vi "Write Prev CCD Config.vi"(8 "error in (no error)":errorcluster, 10 "Prev CCD Config":T1={"PREAMP"=0, "READOUT_RATE"=0, "EM_GAIN"=2, "VERTICAL_SHIFT_SPEED"=0, "READ_MODE"=4, "FRAME_TRANSFER"=TRUE, "VERTICAL_CLOCK_VOLTAGE"=0, "ACQUISITION_MODE"=2, "AD_CHANNEL"=0, "EM_MODE"=0, "SHUTTER_TTL"=0, "SHUTTER_OPENING_TIME"=50, "SHUTTER_CLOSING_TIME"=50, "SHUTTER_MODE"=2, "TRIGGER_MODE"=0, "VBIN"=1, "INITIAL_LINE"=1, "INITIAL_COLUMN"=1, "FINAL_LINE"=1024, "FINAL_COLUMN"=1024, "HBIN"=1} {"TRIGGER_MODE" items=["Internal", "External", "N/A", "N/A_1", "N/A_2", "N/A_3", "External Start"]; "SHUTTER_MODE" items=["Auto", "Open", "Closed"]; "SHUTTER_TTL" items=["TTL Low", "TTL High"]; "EM_MODE" items=["Electron Multiplying", "Conventional"]; "ACQUISITION_MODE" items=["Single", "Accumulate", "Kinetic"]; "VERTICAL_CLOCK_VOLTAGE" items=["0", "+1", "+2", "+3", "+4"]; "READ_MODE" items=["Full Vertical Binning", "Multi-track", "Random-track", "Single-track", "Image"]; "VERTICAL_SHIFT_SPEED" items=["0.6", "1.13", "2.2", "4.33"]; "READOUT_RATE" items=["1 MHz", "0.1 MHz"]; "PREAMP" items=["Gain 1", "Gain 2"]}, 11 "Simulated_CCD_Camera in":refnum<class "Simulated Camera.lvclass">) -> (0 "error out":errorcluster, 3 "Simulated_CCD_Camera out":refnum<class "Simulated Camera.lvclass">)   [LabVIEW 2018, in "Simulated Camera.lvclass"]
uses:
  Simulated Camera.lvclass
  Simulated Camera.lvclass/Simulated Camera.ctl
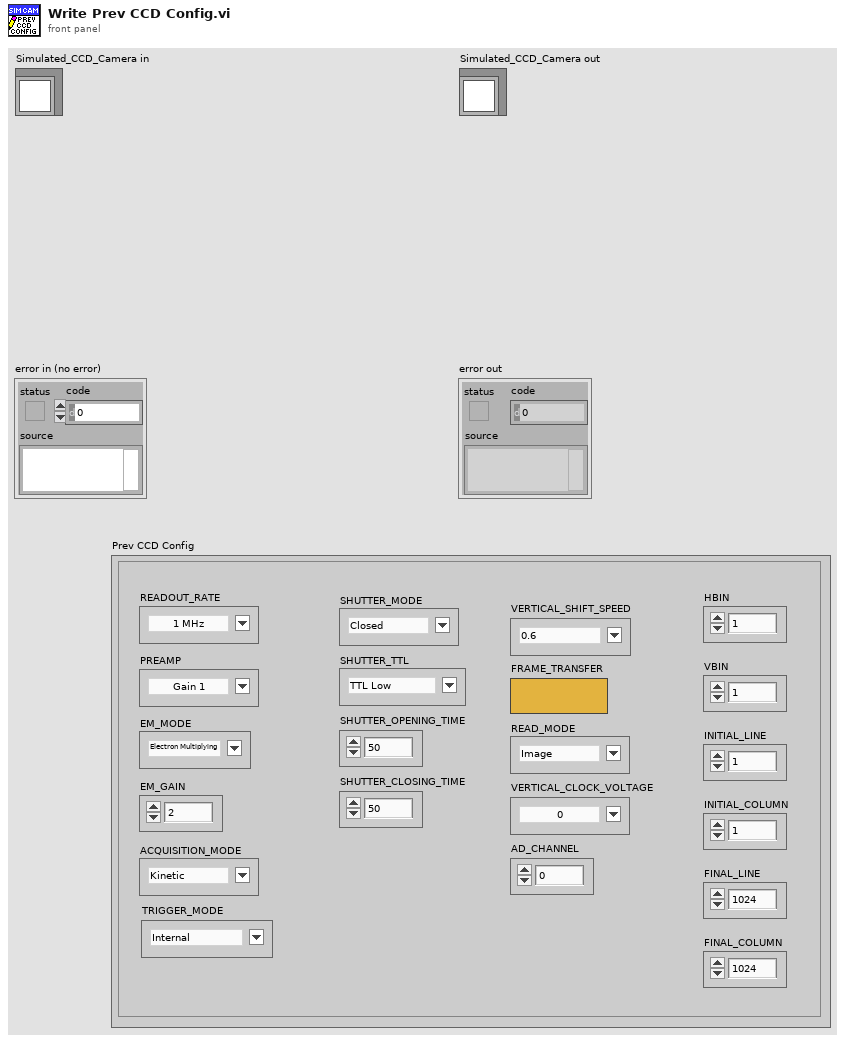
[diagram p1: front panel]
types:
  T1 = cluster{"PREAMP":u16, "READOUT_RATE":u16, "EM_GAIN":u16, "VERTICAL_SHIFT_SPEED":u16, "READ_MODE":u16, "FRAME_TRANSFER":bool, "VERTICAL_CLOCK_VOLTAGE":u16, "ACQUISITION_MODE":u16, "AD_CHANNEL":u16, "EM_MODE":u16, "SHUTTER_TTL":u16, "SHUTTER_OPENING_TIME":u16, "SHUTTER_CLOSING_TIME":u16, "SHUTTER_MODE":u16, "TRIGGER_MODE":u16, "VBIN":u16, "INITIAL_LINE":u16, "INITIAL_COLUMN":u16, "FINAL_LINE":u16, "FINAL_COLUMN":u16, "HBIN":u16}
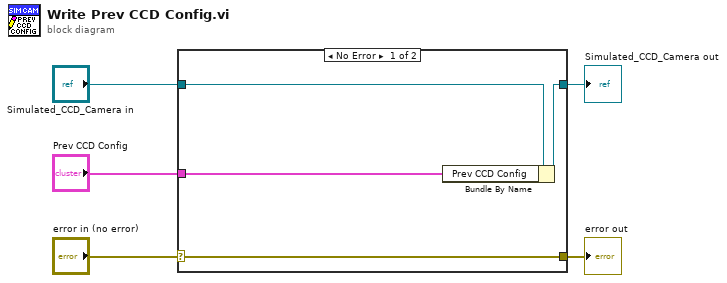
[diagram p0: block diagram]
diagram:
  n1 = case shown="No Error" "error in (no error)" {
    selector: "error in (no error)" -> [w9 w10]
    tunnel: [w9 w10] -> w4
    tunnel: [w7 w11] -> w2
    tunnel: "Simulated_CCD_Camera in" -> [w8 w11]
    tunnel: "Prev CCD Config" -> [w6 _]
    frame No Error {
      n2 = Bundle By Name(cluster=w8, "Prev CCD Config"=w6) -> (w7:refnum<class "Simulated Camera.lvclass">)
    }
    frame Error {
    }
  }
  "error out" <- w4
  "Simulated_CCD_Camera out" <- w2
